vi "Lab Panel V4.85.vi"() -> ()   [LabVIEW 2013] (continued)
                            n2235 = Bundle(cluster=w4040, "amps"=w4044, "volts"=w4043, "pf"=w4042) -> (w4041:cluster{"amps":dbl, "volts":dbl, "pf":dbl})
                            n2236 = local write "ON L05-1"(w4041) -> ()
                          }
                        }
                      }
                      frame #1 {
                        n2237 = Unbundle(w4049) -> ("amps"=w4048:dbl, "volts"=w4047:dbl, "pf"=w4046:dbl)
                        n2238 = case shown="True" w4050 {
                          tunnel: w4057 -> [_ w4089]
                          tunnel: w4056 -> [_ w4096]
                          tunnel: w4055 -> [_ _]
                          tunnel: w4054 -> [_ _]
                          tunnel: w4053 -> [_ w4095]
                          tunnel: w4052 -> [_ w4094]
                          tunnel: w4051 -> [_ w4059]
                          tunnel: w4048 -> [_ w4091]
                          tunnel: w4047 -> [_ w4090]
                          tunnel: w4046 -> [_ w4088]
                          tunnel: w4045 -> [_ w4080]
                          frame False {
                          }
                          frame True {
                            n2239 = local read "TDMS LAB05-1"() -> (w4093:refnum<k34>)
                            n2240 = Build Array(w4090) -> (w4085:dbl[])
                            n2241 = Build Array(w4088) -> (w4084:dbl[])
                            n2242 = Build Array(w4095) -> (w4083:dbl[])
                            n2243 = Build Array(w4096) -> (w4082:dbl[])
                            n2244 = Build Array(w4091) -> (w4087:dbl[])
                            n2245 = Build Array(w4089) -> (w4086:dbl[])
                            n2246 = Build Array(w4094) -> (w4081:dbl[])
                            n2247 = Build Array("AMPS ON", "AMPS OFF", "VOLTS", "PF", "TEMP Live", "TEMP Neut", "CYCLE") -> (w4064:string[])
                            n2248 = Bundle By Name("Y"=w4087, "t0"=w4080) -> (w4079:waveform(dbl))  [unwired: 1 in]
                            n2249 = Bundle By Name("Y"=w4086, "t0"=w4080) -> (w4078:waveform(dbl))  [unwired: 1 in]
                            n2250 = Bundle By Name("Y"=w4085, "t0"=w4080) -> (w4077:waveform(dbl))  [unwired: 1 in]
                            n2251 = Bundle By Name("Y"=w4084, "t0"=w4080) -> (w4076:waveform(dbl))  [unwired: 1 in]
                            n2252 = Bundle By Name("Y"=w4083, "t0"=w4080) -> (w4075:waveform(dbl))  [unwired: 1 in]
                            n2253 = Bundle By Name("Y"=w4082, "t0"=w4080) -> (w4074:waveform(dbl))  [unwired: 1 in]
                            n2254 = Bundle By Name("Y"=w4081, "t0"=w4080) -> (w4073:waveform(dbl))  [unwired: 1 in]
                            n2255 = Build Array(w4079, w4078, w4077, w4076, w4075, w4074, w4073) -> (w4072:waveform(dbl)[])
                            n2256 = TDMS Write(0:w4093, 5:"TEST VALUES", 7:w4064, 9:w4072) -> (4:w4063:refnum<k34>, 6:w4062:string, 15:w4061:errorcluster)  [unwired: 2 in, 1 out]
                            n2257 = TDMS Write(0:w4063, 5:w4062, 7:"TIME", 9:w4059, 11:w4061) -> (15:w4058:errorcluster)  [unwired: 1 in, 3 out]
                            n2258 = local write "data file error"(w4058) -> ()
                          }
                        }
                      }
                    }
                  }
                }
              }
              frame #9 {
                n2259 = case shown="True" w4097 {
                  tunnel: w4101 -> [_ w4106]
                  tunnel: w4100 -> [_ w4105]
                  tunnel: w4099 -> [_ w4103]
                  tunnel: w4098 -> [_ w4102]
                  frame False {
                  }
                  frame True {
                    n2260 = local read "DISP LAB05-2"() -> (w4107:T4)
                    n2261 = local read "SIG LAB05-2"() -> (w4108:T2)
                    n2262 = local read "ON L05-2"() -> (w4104:cluster{"amps":dbl, "volts":dbl, "pf":dbl})
                    n2263 = Unbundle(w4108) -> ("AMPS"=w4114:dbl, "VOLTS"=w4112:dbl, "PF"=w4111:dbl, "Tmp Live"=w4110:dbl, "Tmp Neut"=w4113:dbl)
                    n2264 = Unbundle(w4107) -> ("CYCLE"=w4109:dbl)  [unwired: 2 out]
                    n2265 = stacked-sequence {
                      tunnel: w4114 -> [w4118 w4137]
                      tunnel: w4113 -> [_ w4136]
                      tunnel: w4112 -> [w4117 w4135]
                      tunnel: w4111 -> [w4116 w4134]
                      tunnel: w4110 -> [_ w4133]
                      tunnel: w4109 -> [_ w4132]
                      tunnel: w4106 -> [_ w4131]
                      tunnel: w4105 -> [w4119 _]
                      tunnel: w4104 -> [w4115 w4129]
                      tunnel: w4103 -> [_ w4130]
                      tunnel: w4102 -> [_ w4125]
                      frame #0 {
                        n2266 = case shown="True" w4119 {
                          tunnel: w4118 -> [_ w4124]
                          tunnel: w4117 -> [_ w4123]
                          tunnel: w4116 -> [_ w4122]
                          tunnel: w4115 -> [_ w4120]
                          frame False {
                          }
                          frame True {
                            n2267 = Bundle(cluster=w4120, "amps"=w4124, "volts"=w4123, "pf"=w4122) -> (w4121:cluster{"amps":dbl, "volts":dbl, "pf":dbl})
                            n2268 = local write "ON L05-2"(w4121) -> ()
                          }
                        }
                      }
                      frame #1 {
                        n2269 = Unbundle(w4129) -> ("amps"=w4128:dbl, "volts"=w4127:dbl, "pf"=w4126:dbl)
                        n2270 = case shown="True" w4130 {
                          tunnel: w4137 -> [_ w4169]
                          tunnel: w4136 -> [_ w4176]
                          tunnel: w4135 -> [_ _]
                          tunnel: w4134 -> [_ _]
                          tunnel: w4133 -> [_ w4175]
                          tunnel: w4132 -> [_ w4174]
                          tunnel: w4131 -> [_ w4139]
                          tunnel: w4128 -> [_ w4171]
                          tunnel: w4127 -> [_ w4170]
                          tunnel: w4126 -> [_ w4168]
                          tunnel: w4125 -> [_ w4160]
                          frame False {
                          }
                          frame True {
                            n2271 = local read "TDMS LAB05-2"() -> (w4173:refnum<k34>)
                            n2272 = Build Array(w4170) -> (w4165:dbl[])
                            n2273 = Build Array(w4168) -> (w4164:dbl[])
                            n2274 = Build Array(w4175) -> (w4163:dbl[])
                            n2275 = Build Array(w4176) -> (w4162:dbl[])
                            n2276 = Build Array(w4171) -> (w4167:dbl[])
                            n2277 = Build Array(w4169) -> (w4166:dbl[])
                            n2278 = Build Array(w4174) -> (w4161:dbl[])
                            n2279 = Build Array("AMPS ON", "AMPS OFF", "VOLTS", "PF", "TEMP Live", "TEMP Neut", "CYCLE") -> (w4144:string[])
                            n2280 = Bundle By Name("Y"=w4167, "t0"=w4160) -> (w4159:waveform(dbl))  [unwired: 1 in]
                            n2281 = Bundle By Name("Y"=w4166, "t0"=w4160) -> (w4158:waveform(dbl))  [unwired: 1 in]
                            n2282 = Bundle By Name("Y"=w4165, "t0"=w4160) -> (w4157:waveform(dbl))  [unwired: 1 in]
                            n2283 = Bundle By Name("Y"=w4164, "t0"=w4160) -> (w4156:waveform(dbl))  [unwired: 1 in]
                            n2284 = Bundle By Name("Y"=w4163, "t0"=w4160) -> (w4155:waveform(dbl))  [unwired: 1 in]
                            n2285 = Bundle By Name("Y"=w4162, "t0"=w4160) -> (w4154:waveform(dbl))  [unwired: 1 in]
                            n2286 = Bundle By Name("Y"=w4161, "t0"=w4160) -> (w4153:waveform(dbl))  [unwired: 1 in]
                            n2287 = Build Array(w4159, w4158, w4157, w4156, w4155, w4154, w4153) -> (w4152:waveform(dbl)[])
                            n2288 = TDMS Write(0:w4173, 5:"TEST VALUES", 7:w4144, 9:w4152) -> (4:w4143:refnum<k34>, 6:w4142:string, 15:w4141:errorcluster)  [unwired: 2 in, 1 out]
                            n2289 = TDMS Write(0:w4143, 5:w4142, 7:"TIME", 9:w4139, 11:w4141) -> (15:w4138:errorcluster)  [unwired: 1 in, 3 out]
                            n2290 = local write "data file error"(w4138) -> ()
                          }
                        }
                      }
                    }
                  }
                }
              }
            }
          }
          frame #13 {
            # "display test values on chart"
            n2291 = disable-structure shown="Disabled" {
              frame Disabled {
                n2292 = case shown="\"ON CYCLE\", Default" "Select  Cycle" {
                  tunnel: [1 _] -> _
                  frame "ON CYCLE", Default {
                  }
                  frame "OFF CYCLE" {
                  }
                }
              }
              frame Enabled {
              }
            }
            n2293 = local read "jig cycle"() -> (w4181:dbl)
            n2294 = local read "on loops"() -> (w4183:dbl)
            n2295 = Add(x=w4183, y=2) -> (x+y=w4180:dbl)
            n2296 = Equal?(x=w4181, y=1) -> (x = y?=w4179:bool)
            n2297 = Equal?(x=w4181, y=w4180) -> (x = y?=w4178:bool)
            n2298 = Or(x=w4179, y=w4178) -> (x .or. y?=w4177:bool)
            "graph flag" <- w4177
            n2299 = global write "Global display 3.vi" "graph flag"(w4177) -> ()
            n2300 = case shown="True" w4177 {
              frame False {
              }
              frame True {
                n2301 = local read "SIG LAB05-1"() -> (w4228:T2)
                n2302 = local read "SIG LAB04-2"() -> (w4229:T2)
                n2303 = local read "SIG LAB05-2"() -> (w4227:T2)
                n2304 = local read "SIG LAB04-1"() -> (w4230:T2)
                n2305 = local read "SIG LAB03-1"() -> (w4232:T2)
                n2306 = local read "SIG LAB03-2"() -> (w4231:T2)
                n2307 = local read "SIG LAB01-1"() -> (w4236:T2)
                n2308 = local read "SIG LAB02-2"() -> (w4233:T2)
                n2309 = local read "SIG LAB02-1"() -> (w4234:T2)
                n2310 = local read "SIG LAB01-2"() -> (w4235:T2)
                n2311 = Unbundle(w4229) -> ("AMPS"=w4219:dbl, "VOLTS"=w4209:dbl, "Tmp Live"=w4199:dbl, "Tmp Neut"=w4189:dbl)  [unwired: 1 out]
                n2312 = Unbundle(w4228) -> ("AMPS"=w4218:dbl, "VOLTS"=w4208:dbl, "Tmp Live"=w4198:dbl, "Tmp Neut"=w4188:dbl)  [unwired: 1 out]
                n2313 = Unbundle(w4227) -> ("AMPS"=w4217:dbl, "VOLTS"=w4207:dbl, "Tmp Live"=w4197:dbl, "Tmp Neut"=w4187:dbl)  [unwired: 1 out]
                n2314 = Unbundle(w4230) -> ("AMPS"=w4220:dbl, "VOLTS"=w4210:dbl, "Tmp Live"=w4200:dbl, "Tmp Neut"=w4190:dbl)  [unwired: 1 out]
                n2315 = Unbundle(w4231) -> ("AMPS"=w4221:dbl, "VOLTS"=w4211:dbl, "Tmp Live"=w4201:dbl, "Tmp Neut"=w4191:dbl)  [unwired: 1 out]
                n2316 = Unbundle(w4232) -> ("AMPS"=w4222:dbl, "VOLTS"=w4212:dbl, "Tmp Live"=w4202:dbl, "Tmp Neut"=w4192:dbl)  [unwired: 1 out]
                n2317 = Unbundle(w4233) -> ("AMPS"=w4223:dbl, "VOLTS"=w4213:dbl, "Tmp Live"=w4203:dbl, "Tmp Neut"=w4193:dbl)  [unwired: 1 out]
                n2318 = Unbundle(w4234) -> ("AMPS"=w4224:dbl, "VOLTS"=w4214:dbl, "Tmp Live"=w4204:dbl, "Tmp Neut"=w4194:dbl)  [unwired: 1 out]
                n2319 = Unbundle(w4236) -> ("AMPS"=w4226:dbl, "VOLTS"=w4216:dbl, "Tmp Live"=w4206:dbl, "Tmp Neut"=w4196:dbl)  [unwired: 1 out]
                n2320 = Unbundle(w4235) -> ("AMPS"=w4225:dbl, "VOLTS"=w4215:dbl, "Tmp Live"=w4205:dbl, "Tmp Neut"=w4195:dbl)  [unwired: 1 out]
                n2321 = stacked-sequence {
                  tunnel: w4226 -> [w4247 _ _ _ _]
                  tunnel: w4225 -> [w4246 _ _ _ _]
                  tunnel: w4224 -> [w4245 _ _ _ _]
                  tunnel: w4223 -> [w4244 _ _ _ _]
                  tunnel: w4222 -> [w4243 _ _ _ _]
                  tunnel: w4221 -> [w4242 _ _ _ _]
                  tunnel: w4220 -> [w4241 _ _ _ _]
                  tunnel: w4219 -> [w4240 _ _ _ _]
                  tunnel: w4218 -> [w4239 _ _ _ _]
                  tunnel: w4217 -> [w4238 _ _ _ _]
                  tunnel: w4216 -> [_ w4258 _ _ _]
                  tunnel: w4215 -> [_ w4257 _ _ _]
                  tunnel: w4214 -> [_ w4256 _ _ _]
                  tunnel: w4213 -> [_ w4255 _ _ _]
                  tunnel: w4212 -> [_ w4254 _ _ _]
                  tunnel: w4211 -> [_ w4253 _ _ _]
                  tunnel: w4210 -> [_ w4252 _ _ _]
                  tunnel: w4209 -> [_ w4251 _ _ _]
                  tunnel: w4208 -> [_ w4250 _ _ _]
                  tunnel: w4207 -> [_ w4249 _ _ _]
                  tunnel: w4206 -> [_ _ w4269 _ _]
                  tunnel: w4205 -> [_ _ w4268 _ _]
                  tunnel: w4204 -> [_ _ w4267 _ _]
                  tunnel: w4203 -> [_ _ w4266 _ _]
                  tunnel: w4202 -> [_ _ w4265 _ _]
                  tunnel: w4201 -> [_ _ w4264 _ _]
                  tunnel: w4200 -> [_ _ w4263 _ _]
                  tunnel: w4199 -> [_ _ w4262 _ _]
                  tunnel: w4198 -> [_ _ w4261 _ _]
                  tunnel: w4197 -> [_ _ w4260 _ _]
                  tunnel: w4196 -> [_ _ _ w4280 _]
                  tunnel: w4195 -> [_ _ _ w4279 _]
                  tunnel: w4194 -> [_ _ _ w4278 _]
                  tunnel: w4193 -> [_ _ _ w4277 _]
                  tunnel: w4192 -> [_ _ _ w4276 _]
                  tunnel: w4191 -> [_ _ _ w4275 _]
                  tunnel: w4190 -> [_ _ _ w4274 _]
                  tunnel: w4189 -> [_ _ _ w4273 _]
                  tunnel: w4188 -> [_ _ _ w4272 _]
                  tunnel: w4187 -> [_ _ _ w4271 _]
                  frame #0 {
                    n2322 = Merge Signals(w4247, w4246, w4245, w4244, w4243, w4242, w4241, w4240, w4239, w4238) -> (→"TEST AMPS CHART":dynamicdata)
                  }
                  frame #1 {
                    n2323 = Merge Signals(w4258, w4257, w4256, w4255, w4254, w4253, w4252, w4251, w4250, w4249) -> (→"TEST VOLTS CHART":dynamicdata)
                  }
                  frame #2 {
                    n2324 = Merge Signals(w4269, w4268, w4267, w4266, w4265, w4264, w4263, w4262, w4261, w4260) -> (→"TEMPERATURE (L) CHART":dynamicdata)
                  }
                  frame #3 {
                    n2325 = Merge Signals(w4280, w4279, w4278, w4277, w4276, w4275, w4274, w4273, w4272, w4271) -> (→"TEMPERATURE (N) CHART":dynamicdata)
                  }
                  frame #4 {
                    n2326 = local read "TEMPERATURE (N) CHART"() -> (w4281:dynamicdata)
                    n2327 = local read "TEMPERATURE (L) CHART"() -> (w4282:dynamicdata)
                    n2328 = local read "TEST VOLTS CHART"() -> (w4283:dynamicdata)
                    n2329 = local read "TEST AMPS CHART"() -> (w4284:dynamicdata)
                    n2330 = global write "Global display 3.vi" "graph temp N"(w4281) -> ()
                    n2331 = global write "Global display 3.vi" "graph temp L"(w4282) -> ()
                    n2332 = global write "Global display 3.vi" "graph volts"(w4283) -> ()
                    n2333 = global write "Global display 3.vi" "graph amps"(w4284) -> ()
                  }
                }
              }
            }
          }
          frame #14 {
            # "check for amps fail"
            # "check for cycle test & temperature rise fail conditions"
            n2334 = local read "on loops"() -> (w4311:dbl)
            n2335 = local read "jig cycle"() -> (w4308:dbl)
            n2336 = local read "jig cycle"() -> (w4313:dbl)
            n2337 = Add(x=w4311, y=3.0) -> (x+y=w4309:dbl)
            n2338 = Equal?(x=w4308, y=w4309) -> (x = y?=w4304:bool)
            n2339 = local read "Fail Loops"() -> (w4285:dbl)
            n2340 = Equal?(x=w4313, y=1.0) -> (x = y?=w4306:bool)
            n2341 = global write "Global 1.vi" "fail count"(w4285) -> ()
            n2342 = stacked-sequence {
              tunnel: w4307 -> [w4316 _ _ _ _ _ _ _ _ _]
              tunnel: w4306 -> [w4317 w4337 w4357 w4377 w4397 w4417 w4437 w4457 w4477 w4497]
              tunnel: w4305 -> [w4314 _ _ _ _ _ _ _ _ _]
              tunnel: w4304 -> [w4315 w4336 w4356 w4376 w4396 w4416 w4436 w4456 w4476 w4496]
              tunnel: w4303 -> [_ w4335 _ _ _ _ _ _ _ _]
              tunnel: w4302 -> [_ w4334 _ _ _ _ _ _ _ _]
              tunnel: w4301 -> [_ _ w4355 _ _ _ _ _ _ _]
              tunnel: w4300 -> [_ _ w4354 _ _ _ _ _ _ _]
              tunnel: w4299 -> [_ _ _ w4375 _ _ _ _ _ _]
              tunnel: w4298 -> [_ _ _ w4374 _ _ _ _ _ _]
              tunnel: w4297 -> [_ _ _ _ w4395 _ _ _ _ _]
              tunnel: w4296 -> [_ _ _ _ w4394 _ _ _ _ _]
              tunnel: w4295 -> [_ _ _ _ _ w4415 _ _ _ _]
              tunnel: w4294 -> [_ _ _ _ _ w4414 _ _ _ _]
              tunnel: w4293 -> [_ _ _ _ _ _ w4435 _ _ _]
              tunnel: w4292 -> [_ _ _ _ _ _ w4434 _ _ _]
              tunnel: w4291 -> [_ _ _ _ _ _ _ w4455 _ _]
              tunnel: w4290 -> [_ _ _ _ _ _ _ w4454 _ _]
              tunnel: w4289 -> [_ _ _ _ _ _ _ _ w4475 _]
              tunnel: w4288 -> [_ _ _ _ _ _ _ _ w4474 _]
              tunnel: w4287 -> [_ _ _ _ _ _ _ _ _ w4495]
              tunnel: w4286 -> [_ _ _ _ _ _ _ _ _ w4494]
              frame #0 {
                # "LAB01-1"
                n2343 = case shown="True" w4314 {
                  tunnel: w4317 -> [_ w4330]
                  tunnel: w4316 -> [_ w4327]
                  tunnel: w4315 -> [_ w4326]
                  frame False {
                  }
                  frame True {
                    n2344 = local read "TEMP START LAB01-1"() -> (w4332:cluster{"TL":dbl, "TN":dbl})
                    n2345 = local read "RESULT LAB01-1"() -> (w4321:bool)
                    n2346 = local read "FAIL LAB01-1"() -> (w4324:cluster{"LO":dbl, "HI":dbl})
                    n2347 = local read "TDMS LAB01-1"() -> (w4331:refnum<k34>)
                    n2348 = local read "SET LAB01-1"() -> (w4328:T5)
                    n2349 = local read "DISP LAB01-1"() -> (w4329:T4)
                    n2350 = local read "SIG LAB01-1"() -> (w4333:T2)
                    n2351 = Bundle("FAIL LAB01-1"=w4324, "SIG LAB01-1"=w4333, "TEMP START LAB01-1"=w4332, "DISP LAB01-1"=w4329, "SET LAB01-1"=w4328, "TDMS LAB01-1"=w4331) -> (w4318:T29)  [unwired: 1 in]
                    n2352 = call "sub vi - cycle&temp fail v6.vi"("Amps Lo?"=w4330, "Input Cluster"=w4318, "SELECT"=w4327, "Amps Hi?"=w4326, "Result In"=w4321) -> ("(FAIL) out"=w4323:cluster{"FAIL LO":dbl, "FAIL HI":dbl}, "(DISP) out"=w4319:T4, "T-RISE"=w4320:cluster{"T-RISE (L)":dbl, "T-RISE (N)":dbl}, "Result Out"=w4322:bool, "file error"=w4325:errorcluster)  [unwired: 10 in]
                    n2353 = local write "TEMP RISE LAB01-1"(w4320) -> ()
                    n2354 = local write "FAIL LAB01-1"(w4323) -> ()
                    n2355 = local write "DISP LAB01-1"(w4319) -> ()
                    n2356 = local write "RESULT LAB01-1"(w4322) -> ()
                    n2357 = local write "data file error"(w4325) -> ()
                  }
                }
              }
              frame #1 {
                # "LAB01-2"
                n2358 = case shown="True" w4335 {
                  tunnel: w4337 -> [_ w4350]
                  tunnel: w4334 -> [_ w4347]
                  tunnel: w4336 -> [_ w4346]
                  frame False {
                  }
                  frame True {
                    n2359 = local read "TEMP START LAB01-2"() -> (w4352:cluster{"TL":dbl, "TN":dbl})
                    n2360 = local read "FAIL LAB01-2"() -> (w4343:cluster{"LO":dbl, "HI":dbl})
                    n2361 = local read "TDMS LAB01-2"() -> (w4351:refnum<k34>)
                    n2362 = local read "SET LAB01-2"() -> (w4348:T5)
                    n2363 = local read "DISP LAB01-2"() -> (w4349:T4)
                    n2364 = local read "RESULT LAB01-2"() -> (w4340:bool)
                    n2365 = local read "SIG LAB01-2"() -> (w4353:T2)
                    n2366 = Bundle("FAIL LAB01-2"=w4343, "SIG LAB01-2"=w4353, "TEMP START LAB01-2"=w4352, "DISP LAB01-2"=w4349, "SET LAB01-2"=w4348, "TDMS LAB01-2"=w4351) -> (w4338:T30)  [unwired: 1 in]
                    n2367 = call "sub vi - cycle&temp fail v6.vi"("Amps Lo?"=w4350, "Input Cluster"=w4338, "SELECT"=w4347, "Amps Hi?"=w4346, "Result In"=w4340) -> ("(FAIL) out"=w4342:cluster{"FAIL LO":dbl, "FAIL HI":dbl}, "(DISP) out"=w4345:T4, "T-RISE"=w4339:cluster{"T-RISE (L)":dbl, "T-RISE (N)":dbl}, "Result Out"=w4341:bool, "file error"=w4344:errorcluster)  [unwired: 10 in]
                    n2368 = local write "TEMP RISE LAB01-2"(w4339) -> ()
                    n2369 = local write "FAIL LAB01-2"(w4342) -> ()
                    n2370 = local write "DISP LAB01-2"(w4345) -> ()
                    n2371 = local write "RESULT LAB01-2"(w4341) -> ()
                    n2372 = local write "data file error"(w4344) -> ()
                  }
                }
              }
              frame #2 {
                # "LAB02-1"
                n2373 = case shown="True" w4355 {
                  tunnel: w4357 -> [_ w4370]
                  tunnel: w4354 -> [_ w4367]
                  tunnel: w4356 -> [_ w4366]
                  frame False {
                  }
                  frame True {
                    n2374 = local read "TEMP START LAB02-1"() -> (w4372:cluster{"TL":dbl, "TN":dbl})
                    n2375 = local read "FAIL LAB02-1"() -> (w4363:cluster{"LO":dbl, "HI":dbl})
                    n2376 = local read "TDMS LAB02-1"() -> (w4371:refnum<k34>)
                    n2377 = local read "SET LAB02-1"() -> (w4368:T5)
                    n2378 = local read "DISP LAB02-1"() -> (w4369:T4)
                    n2379 = local read "SIG LAB02-1"() -> (w4373:T2)
                    n2380 = local read "RESULT LAB02-1"() -> (w4360:bool)
                    n2381 = Bundle("FAIL LAB02-1"=w4363, "SIG LAB02-1"=w4373, "TEMP START LAB02-1"=w4372, "DISP LAB02-1"=w4369, "SET LAB02-1"=w4368, "TDMS LAB02-1"=w4371) -> (w4358:T31)  [unwired: 1 in]
                    n2382 = call "sub vi - cycle&temp fail v6.vi"("Amps Lo?"=w4370, "Input Cluster"=w4358, "SELECT"=w4367, "Amps Hi?"=w4366, "Result In"=w4360) -> ("(FAIL) out"=w4362:cluster{"FAIL LO":dbl, "FAIL HI":dbl}, "(DISP) out"=w4365:T4, "T-RISE"=w4359:cluster{"T-RISE (L)":dbl, "T-RISE (N)":dbl}, "Result Out"=w4361:bool, "file error"=w4364:errorcluster)  [unwired: 10 in]
                    n2383 = local write "TEMP RISE LAB02-1"(w4359) -> ()
                    n2384 = local write "FAIL LAB02-1"(w4362) -> ()
                    n2385 = local write "DISP LAB02-1"(w4365) -> ()
                    n2386 = local write "RESULT LAB02-1"(w4361) -> ()
                    n2387 = local write "data file error"(w4364) -> ()
                  }
                }
              }
              frame #3 {
                # "LAB02-2"
                n2388 = case shown="True" w4375 {
                  tunnel: w4377 -> [_ w4390]
                  tunnel: w4374 -> [_ w4387]
                  tunnel: w4376 -> [_ w4386]
                  frame False {
                  }
                  frame True {
                    n2389 = local read "TEMP START LAB02-2"() -> (w4392:cluster{"TL":dbl, "TN":dbl})
                    n2390 = local read "FAIL LAB02-2"() -> (w4383:cluster{"LO":dbl, "HI":dbl})
                    n2391 = local read "TDMS LAB02-2"() -> (w4391:refnum<k34>)
                    n2392 = local read "SET LAB02-2"() -> (w4388:T5)
                    n2393 = local read "DISP LAB02-2"() -> (w4389:T4)
                    n2394 = local read "SIG LAB02-2"() -> (w4393:T2)
                    n2395 = local read "RESULT LAB02-2"() -> (w4380:bool)
                    n2396 = Bundle("FAIL LAB02-2"=w4383, "SIG LAB02-2"=w4393, "TEMP START LAB02-2"=w4392, "DISP LAB02-2"=w4389, "SET LAB02-2"=w4388, "TDMS LAB02-2"=w4391) -> (w4378:T32)  [unwired: 1 in]
                    n2397 = call "sub vi - cycle&temp fail v6.vi"("Amps Lo?"=w4390, "Input Cluster"=w4378, "SELECT"=w4387, "Amps Hi?"=w4386, "Result In"=w4380) -> ("(FAIL) out"=w4382:cluster{"FAIL LO":dbl, "FAIL HI":dbl}, "(DISP) out"=w4385:T4, "T-RISE"=w4379:cluster{"T-RISE (L)":dbl, "T-RISE (N)":dbl}, "Result Out"=w4381:bool, "file error"=w4384:errorcluster)  [unwired: 10 in]
                    n2398 = local write "TEMP RISE LAB02-2"(w4379) -> ()
                    n2399 = local write "FAIL LAB02-2"(w4382) -> ()
                    n2400 = local write "DISP LAB02-2"(w4385) -> ()
                    n2401 = local write "RESULT LAB02-2"(w4381) -> ()
                    n2402 = local write "data file error"(w4384) -> ()
                  }
                }
              }
              frame #4 {
                # "LAB03-1"
                n2403 = case shown="True" w4395 {
                  tunnel: w4397 -> [_ w4410]
                  tunnel: w4394 -> [_ w4407]
                  tunnel: w4396 -> [_ w4406]
                  frame False {
                  }
                  frame True {
                    n2404 = local read "TEMP START LAB03-1"() -> (w4412:cluster{"TL":dbl, "TN":dbl})
                    n2405 = local read "FAIL LAB03-1"() -> (w4403:cluster{"LO":dbl, "HI":dbl})
                    n2406 = local read "TDMS LAB03-1"() -> (w4411:refnum<k34>)
                    n2407 = local read "SET LAB03-1"() -> (w4408:T5)
                    n2408 = local read "DISP LAB03-1"() -> (w4409:T4)
                    n2409 = local read "SIG LAB03-1"() -> (w4413:T2)
                    n2410 = local read "RESULT LAB03-1"() -> (w4400:bool)
                    n2411 = Bundle("FAIL LAB03-1"=w4403, "SIG LAB03-1"=w4413, "TEMP START LAB03-1"=w4412, "DISP LAB03-1"=w4409, "SET LAB03-1"=w4408, "TDMS LAB03-1"=w4411) -> (w4398:T33)  [unwired: 1 in]
                    n2412 = call "sub vi - cycle&temp fail v6.vi"("Amps Lo?"=w4410, "Input Cluster"=w4398, "SELECT"=w4407, "Amps Hi?"=w4406, "Result In"=w4400) -> ("(FAIL) out"=w4402:cluster{"FAIL LO":dbl, "FAIL HI":dbl}, "(DISP) out"=w4405:T4, "T-RISE"=w4399:cluster{"T-RISE (L)":dbl, "T-RISE (N)":dbl}, "Result Out"=w4401:bool, "file error"=w4404:errorcluster)  [unwired: 10 in]
                    n2413 = local write "TEMP RISE LAB03-1"(w4399) -> ()
                    n2414 = local write "FAIL LAB03-1"(w4402) -> ()
                    n2415 = local write "DISP LAB03-1"(w4405) -> ()
                    n2416 = local write "RESULT LAB03-1"(w4401) -> ()
                    n2417 = local write "data file error"(w4404) -> ()
                  }
                }
              }
              frame #5 {
                # "LAB03-2"
                n2418 = case shown="True" w4415 {
                  tunnel: w4417 -> [_ w4430]
                  tunnel: w4414 -> [_ w4427]
                  tunnel: w4416 -> [_ w4426]
                  frame False {
                  }
                  frame True {
                    n2419 = local read "TEMP START LAB03-2"() -> (w4432:cluster{"TL":dbl, "TN":dbl})
                    n2420 = local read "FAIL LAB03-2"() -> (w4423:cluster{"LO":dbl, "HI":dbl})
                    n2421 = local read "TDMS LAB03-2"() -> (w4431:refnum<k34>)
                    n2422 = local read "SET LAB03-2"() -> (w4428:T5)
                    n2423 = local read "DISP LAB03-2"() -> (w4429:T4)
                    n2424 = local read "RESULT LAB03-2"() -> (w4420:bool)
                    n2425 = local read "SIG LAB03-2"() -> (w4433:T2)
                    n2426 = Bundle("FAIL LAB03-2"=w4423, "SIG LAB03-2"=w4433, "TEMP START LAB03-2"=w4432, "DISP LAB03-2"=w4429, "SET LAB03-2"=w4428, "TDMS LAB03-2"=w4431) -> (w4418:T34)  [unwired: 1 in]
                    n2427 = call "sub vi - cycle&temp fail v6.vi"("Amps Lo?"=w4430, "Input Cluster"=w4418, "SELECT"=w4427, "Amps Hi?"=w4426, "Result In"=w4420) -> ("(FAIL) out"=w4422:cluster{"FAIL LO":dbl, "FAIL HI":dbl}, "(DISP) out"=w4425:T4, "T-RISE"=w4419:cluster{"T-RISE (L)":dbl, "T-RISE (N)":dbl}, "Result Out"=w4421:bool, "file error"=w4424:errorcluster)  [unwired: 10 in]
                    n2428 = local write "FAIL LAB03-2"(w4422) -> ()
                    n2429 = local write "TEMP RISE LAB03-2"(w4419) -> ()
                    n2430 = local write "DISP LAB03-2"(w4425) -> ()
                    n2431 = local write "RESULT LAB03-2"(w4421) -> ()
                    n2432 = local write "data file error"(w4424) -> ()
                  }
                }
              }
              frame #6 {
                # "LAB04-1"
                n2433 = case shown="True" w4435 {
                  tunnel: w4437 -> [_ w4450]
                  tunnel: w4434 -> [_ w4447]
                  tunnel: w4436 -> [_ w4446]
                  frame False {
                  }
                  frame True {
                    n2434 = local read "TEMP START LAB04-1"() -> (w4452:cluster{"TL":dbl, "TN":dbl})
                    n2435 = local read "FAIL LAB04-1"() -> (w4443:cluster{"LO":dbl, "HI":dbl})
                    n2436 = local read "TDMS LAB04-1"() -> (w4451:refnum<k34>)
                    n2437 = local read "SET LAB04-1"() -> (w4448:T5)
                    n2438 = local read "DISP LAB04-1"() -> (w4449:T4)
                    n2439 = local read "SIG LAB04-1"() -> (w4453:T2)
                    n2440 = local read "RESULT LAB04-1"() -> (w4440:bool)
                    n2441 = Bundle("FAIL LAB04-1"=w4443, "SIG LAB04-1"=w4453, "TEMP START LAB04-1"=w4452, "DISP LAB04-1"=w4449, "SET LAB04-1"=w4448, "TDMS LAB04-1"=w4451) -> (w4438:T35)  [unwired: 1 in]
                    n2442 = call "sub vi - cycle&temp fail v6.vi"("Amps Lo?"=w4450, "Input Cluster"=w4438, "SELECT"=w4447, "Amps Hi?"=w4446, "Result In"=w4440) -> ("(FAIL) out"=w4442:cluster{"FAIL LO":dbl, "FAIL HI":dbl}, "(DISP) out"=w4445:T4, "T-RISE"=w4439:cluster{"T-RISE (L)":dbl, "T-RISE (N)":dbl}, "Result Out"=w4441:bool, "file error"=w4444:errorcluster)  [unwired: 10 in]
                    n2443 = local write "TEMP RISE LAB04-1"(w4439) -> ()
                    n2444 = local write "FAIL LAB04-1"(w4442) -> ()
                    n2445 = local write "DISP LAB04-1"(w4445) -> ()
                    n2446 = local write "RESULT LAB04-1"(w4441) -> ()
                    n2447 = local write "data file error"(w4444) -> ()
                  }
                }
              }
              frame #7 {
                # "LAB04-2"
                n2448 = case shown="True" w4455 {
                  tunnel: w4457 -> [_ w4470]
                  tunnel: w4454 -> [_ w4467]
                  tunnel: w4456 -> [_ w4466]
                  frame False {
                  }
                  frame True {
                    n2449 = local read "TEMP START LAB04-2"() -> (w4472:cluster{"TL":dbl, "TN":dbl})
                    n2450 = local read "FAIL LAB04-2"() -> (w4463:cluster{"LO":dbl, "HI":dbl})
                    n2451 = local read "TDMS LAB04-2"() -> (w4471:refnum<k34>)
                    n2452 = local read "SET LAB04-2"() -> (w4468:T5)
                    n2453 = local read "DISP LAB04-2"() -> (w4469:T4)
                    n2454 = local read "SIG LAB04-2"() -> (w4473:T2)
                    n2455 = local read "RESULT LAB04-2"() -> (w4460:bool)
                    n2456 = Bundle("FAIL LAB04-2"=w4463, "SIG LAB04-2"=w4473, "TEMP START LAB04-2"=w4472, "DISP LAB04-2"=w4469, "SET LAB04-2"=w4468, "TDMS LAB04-2"=w4471) -> (w4458:T36)  [unwired: 1 in]
                    n2457 = call "sub vi - cycle&temp fail v6.vi"("Amps Lo?"=w4470, "Input Cluster"=w4458, "SELECT"=w4467, "Amps Hi?"=w4466, "Result In"=w4460) -> ("(FAIL) out"=w4462:cluster{"FAIL LO":dbl, "FAIL HI":dbl}, "(DISP) out"=w4465:T4, "T-RISE"=w4459:cluster{"T-RISE (L)":dbl, "T-RISE (N)":dbl}, "Result Out"=w4461:bool, "file error"=w4464:errorcluster)  [unwired: 10 in]
                    n2458 = local write "TEMP RISE LAB04-2"(w4459) -> ()
                    n2459 = local write "FAIL LAB04-2"(w4462) -> ()
                    n2460 = local write "DISP LAB04-2"(w4465) -> ()
                    n2461 = local write "RESULT LAB04-2"(w4461) -> ()
                    n2462 = local write "data file error"(w4464) -> ()
                  }
                }
              }
              frame #8 {
                # "LAB05-1"
                n2463 = case shown="True" w4475 {
                  tunnel: w4477 -> [_ w4490]
                  tunnel: w4474 -> [_ w4487]
                  tunnel: w4476 -> [_ w4486]
                  frame False {
                  }
                  frame True {
                    n2464 = local read "TEMP START LAB05-1"() -> (w4492:cluster{"TL":dbl, "TN":dbl})
                    n2465 = local read "FAIL LAB05-1"() -> (w4483:cluster{"LO":dbl, "HI":dbl})
                    n2466 = local read "TDMS LAB05-1"() -> (w4491:refnum<k34>)
                    n2467 = local read "SET LAB05-1"() -> (w4488:T5)
                    n2468 = local read "DISP LAB05-1"() -> (w4489:T4)
                    n2469 = local read "SIG LAB05-1"() -> (w4493:T2)
                    n2470 = local read "RESULT LAB05-1"() -> (w4480:bool)
                    n2471 = Bundle("FAIL LAB05-1"=w4483, "SIG LAB05-1"=w4493, "TEMP START LAB05-1"=w4492, "DISP LAB05-1"=w4489, "SET LAB05-1"=w4488, "TDMS LAB05-1"=w4491) -> (w4478:T37)  [unwired: 1 in]
                    n2472 = call "sub vi - cycle&temp fail v6.vi"("Amps Lo?"=w4490, "Input Cluster"=w4478, "SELECT"=w4487, "Amps Hi?"=w4486, "Result In"=w4480) -> ("(FAIL) out"=w4482:cluster{"FAIL LO":dbl, "FAIL HI":dbl}, "(DISP) out"=w4485:T4, "T-RISE"=w4479:cluster{"T-RISE (L)":dbl, "T-RISE (N)":dbl}, "Result Out"=w4481:bool, "file error"=w4484:errorcluster)  [unwired: 10 in]
                    n2473 = local write "TEMP RISE LAB05-1"(w4479) -> ()
                    n2474 = local write "FAIL LAB05-1"(w4482) -> ()
                    n2475 = local write "DISP LAB05-1"(w4485) -> ()
                    n2476 = local write "RESULT LAB05-1"(w4481) -> ()
                    n2477 = local write "data file error"(w4484) -> ()
                  }
                }
              }
              frame #9 {
                # "LAB05-2"
                n2478 = case shown="True" w4495 {
                  tunnel: w4497 -> [_ w4510]
                  tunnel: w4494 -> [_ w4507]
                  tunnel: w4496 -> [_ w4506]
                  frame False {
                  }
                  frame True {
                    n2479 = local read "TEMP START LAB05-2"() -> (w4512:cluster{"TL":dbl, "TN":dbl})
                    n2480 = local read "FAIL LAB05-2"() -> (w4503:cluster{"LO":dbl, "HI":dbl})
                    n2481 = local read "TDMS LAB05-2"() -> (w4511:refnum<k34>)
                    n2482 = local read "SET LAB05-2"() -> (w4508:T5)
                    n2483 = local read "DISP LAB05-2"() -> (w4509:T4)
                    n2484 = local read "SIG LAB05-2"() -> (w4513:T2)
                    n2485 = local read "RESULT LAB05-2"() -> (w4500:bool)
                    n2486 = Bundle("FAIL LAB05-2"=w4503, "SIG LAB05-2"=w4513, "TEMP START LAB05-2"=w4512, "DISP LAB05-2"=w4509, "SET LAB05-2"=w4508, "TDMS LAB05-2"=w4511) -> (w4498:T38)  [unwired: 1 in]
                    n2487 = call "sub vi - cycle&temp fail v6.vi"("Amps Lo?"=w4510, "Input Cluster"=w4498, "SELECT"=w4507, "Amps Hi?"=w4506, "Result In"=w4500) -> ("(FAIL) out"=w4502:cluster{"FAIL LO":dbl, "FAIL HI":dbl}, "(DISP) out"=w4505:T4, "T-RISE"=w4499:cluster{"T-RISE (L)":dbl, "T-RISE (N)":dbl}, "Result Out"=w4501:bool, "file error"=w4504:errorcluster)  [unwired: 10 in]
                    n2488 = local write "TEMP RISE LAB05-2"(w4499) -> ()
                    n2489 = local write "FAIL LAB05-2"(w4502) -> ()
                    n2490 = local write "DISP LAB05-2"(w4505) -> ()
                    n2491 = local write "RESULT LAB05-2"(w4501) -> ()
                    n2492 = local write "data file error"(w4504) -> ()
                  }
                }
              }
            }
          }
          frame #15 {
            # "run calibration routine"
            n2493 = local read "SET (cal)"() -> (w4514:bool)
            n2494 = case shown="True" w4514 {
              frame False {
              }
              frame True {
                n2495 = stacked-sequence {
                  seq-local: [w4515 _ _] -> [_ w4517 _]
                  frame #0 {
                    n2496 = call "CALIBRATION PASSWORD"() -> ("PASSWORD"=w4515:string)  [unwired: 17 in, 2 out]
                  }
                  frame #1 {
                    n2497 = Equal?(x=w4517, y="7777") -> (x = y?=w4516:bool)
                    n2498 = case shown="True" w4516 {
                      frame False {
                      }
                      frame True {
                        n2499 = stacked-sequence {
                          frame #0 {
                            n2500 = call "sub vi - calibration v1.vi"() -> ()  [unwired: 12 in]
                          }
                          frame #1 {
                            n2501 = call "sub vi - get calibration values v1.vi"() -> ("LAB01 (CAL)"=w4523:T12, "LAB02 (CAL)"=w4522:T13, "LAB03 (CAL)"=w4521:T12, "LAB04 (CAL)"=w4520:T12, "calibration file error out"=w4524:errorcluster, "LAB05 (CAL)"=w4519:T12)  [unwired: 10 in]
                            n2502 = local write "cal file error out"(w4524) -> ()
                            n2503 = local write "CAL LAB04"(w4520) -> ()
                            n2504 = local write "CAL LAB05"(w4519) -> ()
                            n2505 = local write "CAL LAB01"(w4523) -> ()
                            n2506 = local write "CAL LAB02"(w4522) -> ()
                            n2507 = local write "CAL LAB03"(w4521) -> ()
                          }
                        }
                      }
                    }
                  }
                  frame #2 {
                    n2508 = local write "SET (cal)"(FALSE) -> ()
                  }
                }
              }
            }
          }
          frame #16 {
            # "save certain settings to file"
            n2509 = String To Path(string="c:\\crabtree\\Set Up\\") -> (path=w4527:path)
            n2510 = Build Path(base path=w4527, name or relative path="settings.bin") -> (appended path=w4529:path)
            n2511 = Build Path(base path=w4527, name or relative path="mail.bin") -> (appended path=w4526:path)
            n2512 = Create Folder(path (use dialog)=w4527) -> (error out=w4532:errorcluster)  [unwired: 2 in, 2 out]
            n2513 = call <vilib>:"Clear Errors.vi"("error in (no error)"=w4532) -> ()  [unwired: 6 in, 1 out]
            n2514 = stacked-sequence {
              seq-local: [w4544 _] -> [_ w4557]
              tunnel: w4529 -> [_ w4558]
              tunnel: w4526 -> [_ w4556]
              frame #0 {
                n2515 = local read "C drive data root dir"() -> (w4543:path)
                n2516 = local read "Select COM port"() -> (w4540:refnum<visa-resource-name>)
                n2517 = local read "Network Directory"() -> (w4549:path)
                n2518 = local read "SET LAB05-2"() -> (w4548:T5)
                n2519 = local read "SET LAB05-1"() -> (w4547:T5)
                n2520 = local read "SET LAB04-2"() -> (w4546:T5)
                n2521 = local read "SET LAB03-2"() -> (w4550:T5)
                n2522 = local read "SET LAB04-1"() -> (w4545:T5)
                n2523 = local read "SET LAB03-1"() -> (w4551:T5)
                n2524 = local read "SET LAB02-2"() -> (w4552:T5)
                n2525 = local read "SET LAB02-1"() -> (w4553:T5)
                n2526 = local read "Temp Delay Lps"() -> (w4539:dbl)
                n2527 = local read "SET LAB01-2"() -> (w4554:T5)
                n2528 = local read "Temp Test Cal"() -> (w4536:dbl)
                n2529 = local read "SET LAB01-1"() -> (w4555:T5)
                n2530 = local read "Temp Value"() -> (w4538:dbl)
                n2531 = local read "Fail Loops"() -> (w4537:dbl)
                n2532 = local read "Test File To"() -> (w4534:string)
                n2533 = local read "spare"() -> (w4535:dbl)
                n2534 = local read "Mail Test Fail"() -> (w4533:bool)
                n2535 = local read "RATE (Hz)"() -> (w4542:dbl)
                n2536 = local read "SAMPLES"() -> (w4541:dbl)
                n2537 = Bundle("SET LAB01-1"=w4555, "SET LAB01-2"=w4554, "SET LAB02-1"=w4553, "SET LAB02-2"=w4552, "SET LAB03-1"=w4551, "SET LAB03-2"=w4550, "SET LAB04-1"=w4545, "SET LAB04-2"=w4546, "SET LAB05-1"=w4547, "SET LAB05-2"=w4548, "Network Directory"=w4549, "C drive data root dir"=w4543, "RATE (Hz)"=w4542, "SAMPLES"=w4541, "Select COM port"=w4540, "Temp Delay Lps"=w4539, "Temp Value"=w4538, "Fail Loops"=w4537, "Temp Test Cal"=w4536, "spare"=w4535, "Test File To"=w4534, "Mail Test Fail"=w4533) -> (w4544:T20)  [unwired: 1 in]
              }
              frame #1 {
                n2538 = event shown="[1] \"SET LAB01-1\", \"SET LAB01-2\", \"SET LAB02-1\", \"SET LAB02-2\", \"SET LAB03-1\", \"SET LAB03-2\", \"SET LAB04-1\", \"SET LAB04-2\", \"SET LAB05-1\", \"SET LAB05-2\", \"Network Directory\", \"C drive data root dir\", \"RATE (Hz)\", \"SAMPLES\", \"Select COM port\", \"Temp Delay Lps\", \"Temp Value\", \"Fail Loops\", \"Temp Test Cal\", \"spare\", \"Test File To\", \"Mail Test Fail\": Value Change" {
                  selector: _ -> [_ _ _]
                  dyn-events: _ -> [_ _ _]
                  timeout: 10.0 -> [_ _ _]
                  tunnel: w4558 -> [_ w4560 _]
                  tunnel: w4557 -> [_ w4561 _]
                  tunnel: w4556 -> [_ _ w4572]
                  event Timeout {
                    n2539 = event-data() -> ()  [unwired: 1 in, 3 out]
                  }
                  event "SET LAB01-1", "SET LAB01-2", "SET LAB02-1", "SET LAB02-2", "SET LAB03-1", "SET LAB03-2", "SET LAB04-1", "SET LAB04-2", "SET LAB05-1", "SET LAB05-2", "Network Directory", "C drive data root dir", "RATE (Hz)", "SAMPLES", "Select COM port", "Temp Delay Lps", "Temp Value", "Fail Loops", "Temp Test Cal", "spare", "Test File To", "Mail Test Fail": Value Change {
                    n2540 = event-data() -> ()  [unwired: 1 in, 6 out]
                    n2541 = Open/Create/Replace File(file path (use dialog)=w4560, operation (0:open)=T19."replace or create") -> (refnum out=w4566:refnum<file>, error out=w4565:errorcluster)  [unwired: 4 in, 1 out]
                    n2542 = Write to Binary File(file (use dialog)=w4566, data=w4561, error in=w4565) -> (refnum out=w4564:refnum<file>, error out=w4563:errorcluster)  [unwired: 3 in, 1 out]
                    n2543 = Close File(refnum=w4564, error in=w4563) -> (error out=w4562:errorcluster)  [unwired: 1 out]
                    n2544 = local write "data file error"(w4562) -> ()
                  }
                  event "MAIL SETTINGS.OUT SERVER ADDRESS", "MAIL SETTINGS.FROM ACCOUNT", "MAIL SETTINGS.USER NAME", "MAIL SETTINGS.PASSWORD", "Auto Mail Send", "TO (string):": Value Change {
                    n2545 = event-data() -> ()  [unwired: 1 in, 6 out]
                    n2546 = local read "MAIL SETTINGS"() -> (w4571:T6)
                    n2547 = local read "Auto Mail Send"() -> (w4569:bool)
                    n2548 = local read "TO (string):"() -> (w4568:string)
                    n2549 = Open/Create/Replace File(file path (use dialog)=w4572, operation (0:open)=T19."replace or create") -> (refnum out=w4577:refnum<file>, error out=w4576:errorcluster)  [unwired: 4 in, 1 out]
                    n2550 = Bundle("MAIL SETTINGS"=w4571, "Auto Mail Send"=w4569, "TO (string):"=w4568) -> (w4570:T39)  [unwired: 1 in]
                    n2551 = Write to Binary File(file (use dialog)=w4577, data=w4570, error in=w4576) -> (refnum out=w4575:refnum<file>, error out=w4574:errorcluster)  [unwired: 3 in, 1 out]
                    n2552 = Close File(refnum=w4575, error in=w4574) -> (error out=w4573:errorcluster)  [unwired: 1 out]
                    n2553 = local write "data file error"(w4573) -> ()
                  }
                }
              }
            }
          }
          frame #17 {
            # "mail control"
            n2554 = local read "MAIL SETTINGS"() -> (w4594:T6)
            n2555 = local read "Auto Mail Send"() -> (w4580:bool)
            n2556 = Unbundle(w4594) -> ("OUT SERVER ADDRESS"=w4593:string, "FROM ACCOUNT"=w4592:string, "TEST MAIL"=w4591:bool)  [unwired: 4 out]
            n2557 = stacked-sequence {
              tunnel: "TO (string):" -> [_ w4633]
              tunnel: w4594 -> [w4599 w4632]
              tunnel: w4593 -> [w4598 w4631]
              tunnel: w4592 -> [w4597 w4630]
              tunnel: w4591 -> [w4596 _]
              tunnel: w4580 -> [_ w4629]
              tunnel: w4590 -> [_ w4628]
              tunnel: w4589 -> [_ w4627]
              tunnel: w4588 -> [_ w4626]
              tunnel: w4587 -> [_ w4625]
              tunnel: w4586 -> [_ w4624]
              tunnel: w4585 -> [_ w4623]
              tunnel: w4584 -> [_ w4622]
              tunnel: w4583 -> [_ w4621]
              tunnel: w4582 -> [_ w4620]
              tunnel: w4581 -> [_ w4619]
              tunnel: "TO (string):" -> [w4595 _]
              frame #0 {
                # "mail test"
                n2558 = case shown="True" w4596 {
                  tunnel: w4599 -> [_ w4603]
                  tunnel: w4595 -> [_ w4602]
                  tunnel: w4598 -> [_ w4601]
                  tunnel: w4597 -> [_ w4600]
                  frame False {
                  }
                  frame True {
                    n2559 = stacked-sequence {
                      seq-local: [_ _ w4613 _] -> [_ _ _ w4614]
                      tunnel: w4603 -> [w4606 _ _ w4618]
                      tunnel: w4602 -> [_ _ w4611 _]
                      tunnel: w4601 -> [_ _ w4609 _]
                      tunnel: w4600 -> [_ _ w4610 _]
                      frame #0 {
                        n2560 = Bundle(cluster=w4606, "TEST MAIL STATUS"="TEST START") -> (w4604:T6)  [unwired: 6 in]
                        n2561 = local write "MAIL SETTINGS"(w4604) -> ()
                      }
                      frame #1 {
                        n2562 = Wait (ms)(milliseconds to wait=500) -> ()  [unwired: 1 out]
                      }
                      frame #2 {
                        n2563 = call "sub vi - send mail v5.vi"("TO:"=w4611, "subject"="MAIL TEST FROM LAB PANEL", "from"=w4610, "out going server"=w4609, "message"="TEST MESSAGE") -> ("error out"=w4613:errorcluster)  [unwired: 10 in]
                      }
                      frame #3 {
                        n2564 = Bundle(cluster=w4618, "TEST MAIL"=FALSE, "TEST MAIL STATUS"="TEST END", "mail error"=w4614) -> (w4616:T6)  [unwired: 4 in]
                        n2565 = local write "MAIL SETTINGS"(w4616) -> ()
                      }
                    }
                  }
                }
              }
              frame #1 {
                # "mail report"
                n2566 = stacked-sequence {
                  seq-local: [_ w4676 _ _] -> [_ _ _ w4866]
                  seq-local: [_ _ w4779 _] -> [_ _ _ w4856]
                  seq-local: [w4643 _ _ _] -> [_ w4693 _ _]
                  seq-local: [w4642 _ _ _] -> [_ w4692 _ _]
                  seq-local: [w4640 _ _ _] -> [_ w4690 _ _]
                  seq-local: [w4641 _ _ _] -> [_ w4691 _ _]
                  seq-local: [w4639 _ _ _] -> [_ w4689 _ _]
                  seq-local: [w4638 _ _ _] -> [_ w4684 _ _]
                  seq-local: [w4637 _ _ _] -> [_ w4685 _ _]
                  seq-local: [w4636 _ _ _] -> [_ w4686 _ _]
                  seq-local: [w4635 _ _ _] -> [_ w4687 _ _]
                  seq-local: [w4634 _ _ _] -> [_ w4688 _ _]
                  tunnel: w4633 -> [_ _ _ w4867]
                  tunnel: w4632 -> [_ _ _ w4850]
                  tunnel: w4631 -> [_ _ _ w4864]
                  tunnel: w4630 -> [_ _ _ w4863]
                  tunnel: w4629 -> [w4674 _ _ w4858]
                  tunnel: w4628 -> [_ _ w4809 _]
                  tunnel: w4627 -> [_ _ w4806 _]
                  tunnel: w4626 -> [_ _ w4805 _]
                  tunnel: w4625 -> [_ _ w4804 _]
                  tunnel: w4624 -> [_ _ w4803 _]
                  tunnel: w4623 -> [_ _ w4802 _]
                  tunnel: w4622 -> [_ _ w4801 _]
                  tunnel: w4621 -> [_ _ w4800 _]
                  tunnel: w4620 -> [_ _ w4799 _]
                  tunnel: w4619 -> [_ _ w4798 _]
                  frame #0 {
                    n2567 = case shown="False" w4674 {
                      frame False {
                        n2568 = local write "mail control"("") -> ()
                      }
                      frame True {
                      }
                    }
                    n2569 = local read "SET LAB01-1"() -> (w4673:T5)
                    n2570 = local read "SET LAB01-2"() -> (w4672:T5)
                    n2571 = local read "SET LAB02-1"() -> (w4671:T5)
                    n2572 = local read "SET LAB02-2"() -> (w4670:T5)
                    n2573 = local read "SET LAB03-1"() -> (w4669:T5)
                    n2574 = local read "SET LAB04-1"() -> (w4667:T5)
                    n2575 = local read "SET LAB05-1"() -> (w4665:T5)
                    n2576 = local read "SET LAB03-2"() -> (w4668:T5)
                    n2577 = local read "SET LAB04-2"() -> (w4666:T5)
                    n2578 = local read "SET LAB05-2"() -> (w4664:T5)
                    n2579 = Unbundle(w4669) -> ("DESCRIPTION"=w4649:string)  [unwired: 4 out]
